vi "HumanActionCache.vi"(4 "Enable Field Oriented Drive":bool, 6 "State":i32, 7 "Rotation":dbl, 8 "Right X":dbl, 9 "Right Y":dbl, 10 "Left X":dbl, 11 "Left Y":dbl) -> (1 "AMotorDemand":dbl, 2 "YMotorDemand":dbl, 3 "XMotorDemand":dbl)   [LabVIEW 2023]
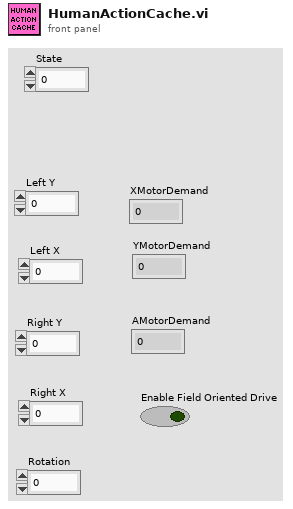
[diagram p1: front panel]
types:
  T1 = enum16{"SpeakerLeft", "SpeakerCenter", "SpeakerRight", "Amp", "Source", "StageLeft", "StageCenter", "StageRight"}
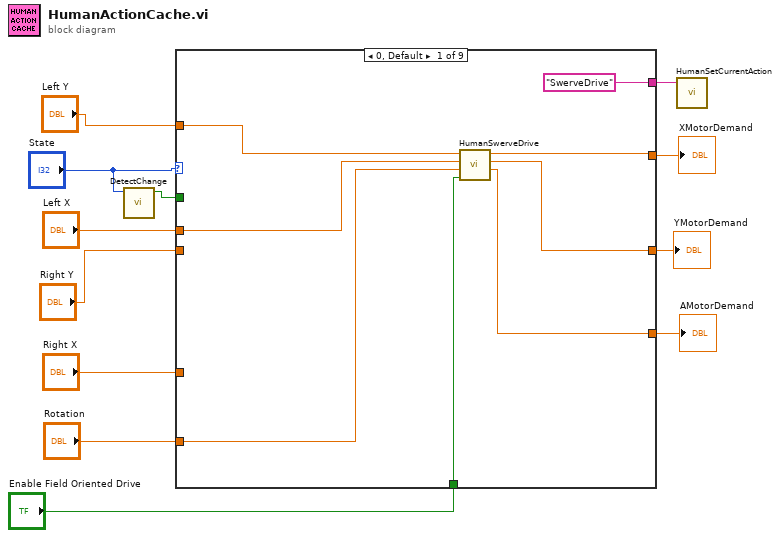
[diagram p0: block diagram]
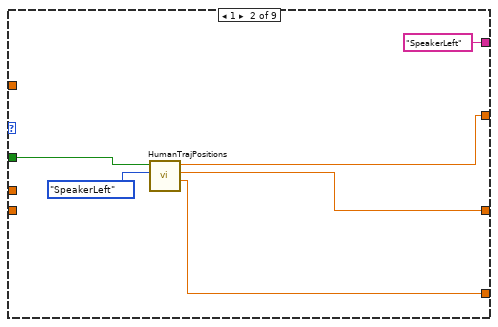
[diagram p2: hidden frame]
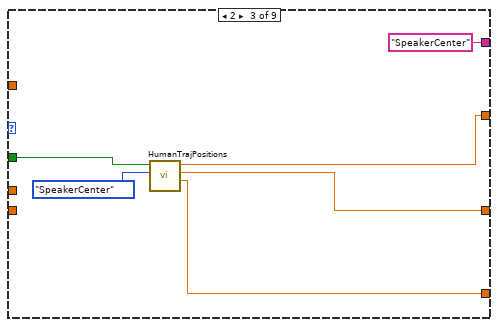
[diagram p3: hidden frame]
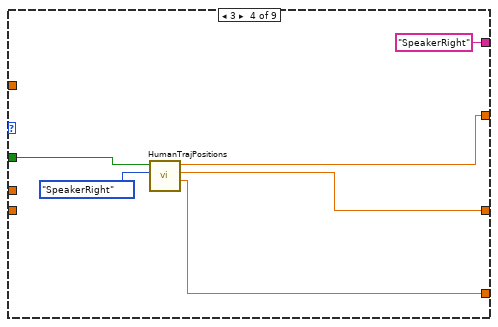
[diagram p4: hidden frame]
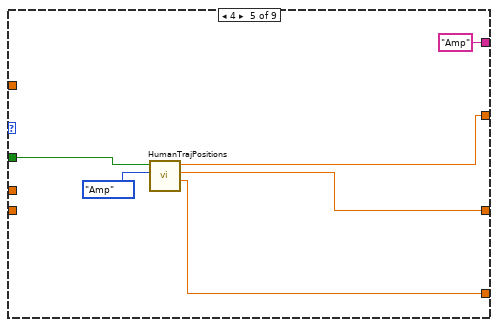
[diagram p5: hidden frame]
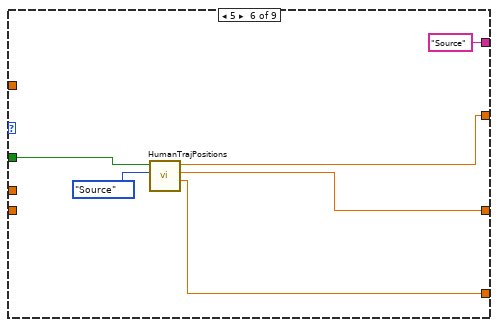
[diagram p6: hidden frame]
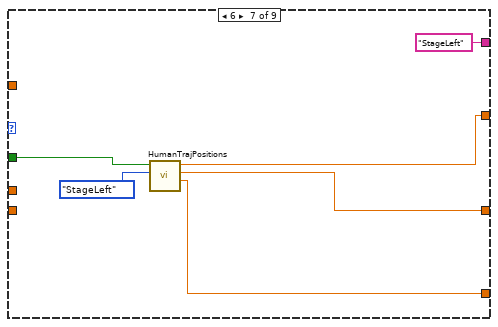
[diagram p7: hidden frame]
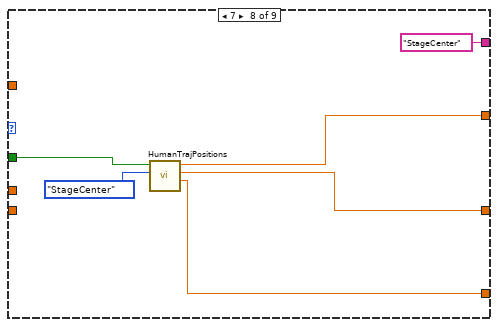
[diagram p8: hidden frame]
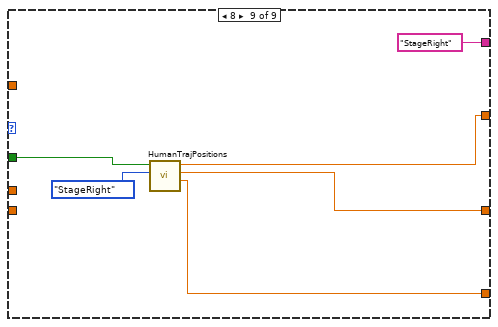
[diagram p9: hidden frame]
diagram:
  n1 = call "DetectChange.vi"("Value"="State") -> ("Changed"=w6:bool)  [unwired: 10 in]
  n2 = case shown="0, Default" "State" {
    tunnel: "Left Y" -> [w19 _ _ _ _ _ _ _ _]
    tunnel: "Right X" -> [_ _ _ _ _ _ _ _ _]
    tunnel: [w16 w25 w31 w37 w43 w49 w55 w61 w67] -> w10
    tunnel: [w15 w24 w30 w36 w42 w48 w54 w60 w66] -> w9
    tunnel: "Right Y" -> [_ _ _ _ _ _ _ _ _]
    tunnel: w6 -> [_ w26 w32 w38 w44 w50 w56 w62 w68]
    tunnel: ["SwerveDrive" "SpeakerLeft" "SpeakerCenter" "SpeakerRight" "Amp" "Source" "StageLeft" "StageCenter" "StageRight"] -> w5
    tunnel: "Left X" -> [w18 _ _ _ _ _ _ _ _]
    tunnel: "Rotation" -> [w17 _ _ _ _ _ _ _ _]
    tunnel: [w14 w23 w29 w35 w41 w47 w53 w59 w65] -> w2
    tunnel: "Enable Field Oriented Drive" -> [w13 _ _ _ _ _ _ _ _]
    frame 0, Default {
      n3 = call "HumanSwerveDrive.vi"("Enable Field Oriented Drive"=w13, "Rotation"=w17, "Y"=w18, "X"=w19) -> ("A"=w14:dbl, "Y"=w15:dbl, "X"=w16:dbl)  [unwired: 5 in]
    }
    frame 1 {
      n4 = call "HumanTrajPositions.vi"("FieldPos"=T1."SpeakerLeft", "Init"=w26) -> ("vAngular"=w23:dbl, "vY"=w24:dbl, "vX"=w25:dbl)  [unwired: 7 in]
    }
    frame 2 {
      n5 = call "HumanTrajPositions.vi"("FieldPos"=T1."SpeakerCenter", "Init"=w32) -> ("vAngular"=w29:dbl, "vY"=w30:dbl, "vX"=w31:dbl)  [unwired: 7 in]
    }
    frame 3 {
      n6 = call "HumanTrajPositions.vi"("FieldPos"=T1."SpeakerRight", "Init"=w38) -> ("vAngular"=w35:dbl, "vY"=w36:dbl, "vX"=w37:dbl)  [unwired: 7 in]
    }
    frame 4 {
      n7 = call "HumanTrajPositions.vi"("FieldPos"=T1."Amp", "Init"=w44) -> ("vAngular"=w41:dbl, "vY"=w42:dbl, "vX"=w43:dbl)  [unwired: 7 in]
    }
    frame 5 {
      n8 = call "HumanTrajPositions.vi"("FieldPos"=T1."Source", "Init"=w50) -> ("vAngular"=w47:dbl, "vY"=w48:dbl, "vX"=w49:dbl)  [unwired: 7 in]
    }
    frame 6 {
      n9 = call "HumanTrajPositions.vi"("FieldPos"=T1."StageLeft", "Init"=w56) -> ("vAngular"=w53:dbl, "vY"=w54:dbl, "vX"=w55:dbl)  [unwired: 7 in]
    }
    frame 7 {
      n10 = call "HumanTrajPositions.vi"("FieldPos"=T1."StageCenter", "Init"=w62) -> ("vAngular"=w59:dbl, "vY"=w60:dbl, "vX"=w61:dbl)  [unwired: 7 in]
    }
    frame 8 {
      n11 = call "HumanTrajPositions.vi"("FieldPos"=T1."StageRight", "Init"=w68) -> ("vAngular"=w65:dbl, "vY"=w66:dbl, "vX"=w67:dbl)  [unwired: 7 in]
    }
  }
  "XMotorDemand" <- w10
  "YMotorDemand" <- w9
  "AMotorDemand" <- w2
  n12 = call "HumanSetCurrentAction.vi"("CurrentState"=w5) -> ()  [unwired: 11 in]
